vi "startContinuousMove.vi"(0 "connection ID in":refnum<k5>, 5 "axis":u8(ring) items=["1", "2", "3"], 7 "start | stop":bool, 9 "direction [t=bwd | f=fwd]":bool, 11 "error in":errorcluster) -> (4 "connection ID":refnum<k5>, 6 "axis_out":u8(ring) items=["1", "2", "3"], 15 "error out":errorcluster)   [LabVIEW 2016]
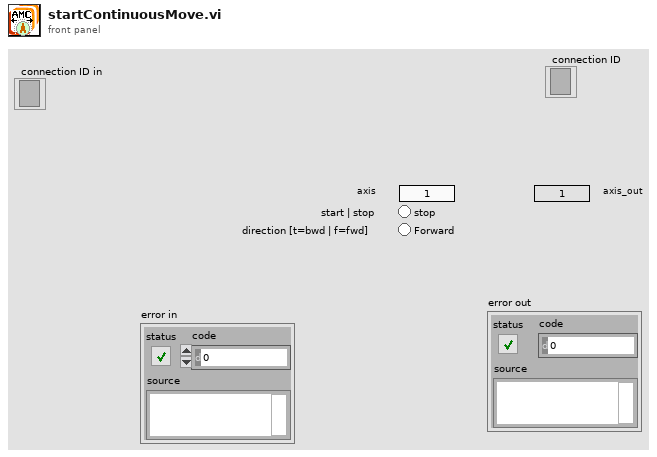
[diagram p1: front panel]
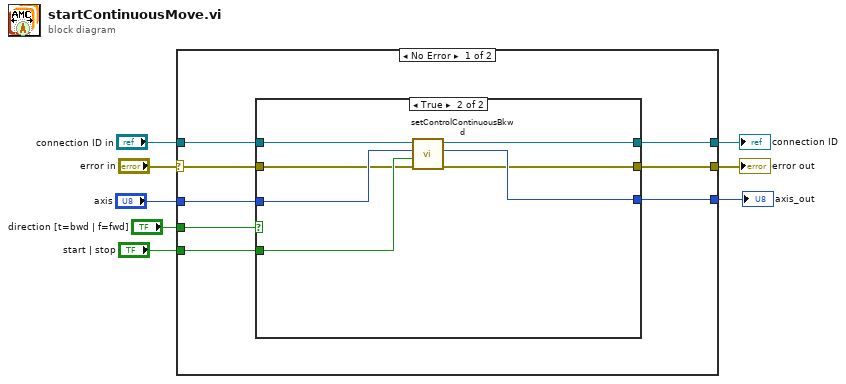
[diagram p0: block diagram]
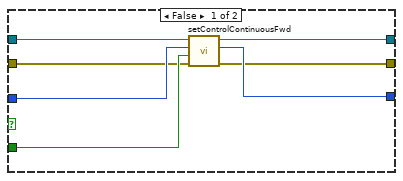
[diagram p2: hidden frame]
diagram:
  n1 = case shown="No Error" "error in" {
    selector: "error in" -> [w10 w32]
    tunnel: [w13 w33] -> w7
    tunnel: "connection ID in" -> [w14 w33]
    tunnel: [w9 w32] -> w5
    tunnel: "direction [t=bwd | f=fwd]" -> [w16 _]
    tunnel: "start | stop" -> [w15 _]
    tunnel: [w11 w31] -> w2
    tunnel: "axis" -> [w12 w31]
    frame No Error {
      n2 = case shown="True" w16 {
        tunnel: w15 -> [w23 w28]
        tunnel: w14 -> [w22 w30]
        tunnel: [w21 w29] -> w13
        tunnel: w12 -> [w20 w27]
        tunnel: [w19 w26] -> w11
        tunnel: w10 -> [w18 w25]
        tunnel: [w17 w24] -> w9
        frame False {
          n3 = call "setControlContinuousFwd.vi"("error in"=w18, "enable"=w23, "axis"=w20, "connection ID"=w22) -> ("error out"=w17:errorcluster, "axis_out"=w19:i32, "connection ID"=w21:refnum<k5>)  [unwired: 5 in]
        }
        frame True {
          n4 = call "setControlContinuousBkwd.vi"("error in"=w25, "enable"=w28, "axis"=w27, "connection ID"=w30) -> ("error out"=w24:errorcluster, "axis_out"=w26:i32, "connection ID"=w29:refnum<k5>)  [unwired: 5 in]
        }
      }
    }
    frame Error {
    }
  }
  "connection ID" <- w7
  "error out" <- w5
  "axis_out" <- w2
